vi "Get Attention Status.vi"(0 "Device ID (0)":i32, 11 "error in (no error)":errorcluster) -> (4 "Device ID out":i32, 6 "TRG_ERROR":bool, 8 "MEM_FULL":bool, 10 "TRG_PASS":bool, 15 "error out":errorcluster)   [LabVIEW 2015, in "KEYENCE LJ-X8000A.lvlib"]
doc: "This function gets the <B>TRG_ERROR</B>/<B>MEM_FULL</B>/<B>TRG_PASS</B> status."
uses:
  KEYENCE LJ-X8000A.lvlib
panel:
  # "(c) 2019 KEYENCE CORPORATION.  ALL RIGHTS RESERVED."
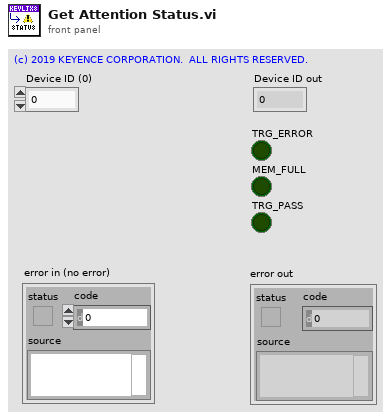
[diagram p1: front panel]
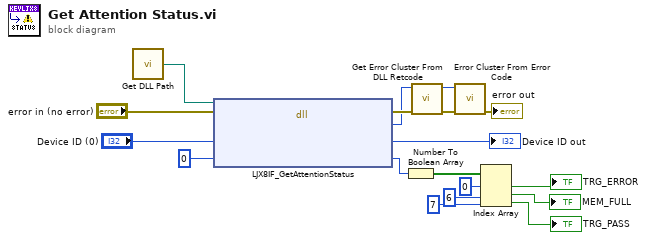
[diagram p0: block diagram]
diagram:
  n1 = call "Get DLL Path.vi"() -> ("DLL Path"=w15:path)  [unwired: 3 in]
  n2 = dll-call lib="C:/Program Files (x86)/National Instruments/LabVIEW 2018/instr.lib/KEYENCE LJ-X8000/LJX8_IF.*" fn="LJX8IF_GetAttentionStatus"(path in=w15, error in="error in (no error)", "lDeviceId"="Device ID (0)", "pwAttentionStatus"=u16 0 ("pnSensorTemperature")) -> (error out=w13:errorcluster, "lRetCode"=w12:i32, "lDeviceId"=→"Device ID out":i32, "pwAttentionStatus"=w6:u16)  [unwired: 1 in, 1 out]
  n3 = Number To Boolean Array(number=w6) -> (Boolean array=w10:bool[])
  n4 = call "Get Error Cluster From DLL Retcode.vi"("error in (no error)"=w13, "DLL Return Code"=w12) -> ("error out"=w14:errorcluster, "VI Error Code"=w1:i32)  [unwired: 8 in]
  n5 = call <vilib>:"Error Cluster From Error Code.vi"("error in (no error)"=w14, "error code (0)"=w1) -> ("error out"=→"error out":errorcluster)  [unwired: 7 in]
  n6 = Index Array(array=w10, index #1=0 ("Žw•W"), index #2=6 ("Žw•W"), index #3=7 ("Žw•W")) -> (element #1=→"TRG_ERROR":bool, element #2=→"MEM_FULL":bool, element #3=→"TRG_PASS":bool)
